vi "LinxI2cOpen.vi"(8 "Error In":errorcluster, 10 "I2C Channel":u8, 11 "LINX Resource":T1) -> (0 "Error Out":errorcluster, 3 "LINX Resource":T1)   [LabVIEW 2014, in "LMH-LINX.lvlib" / "Local IO.lvlib"]
uses:
  <vilib>/MakerHub/LINX/Private/Local IO/Local IO.lvlib
  <vilib>/MakerHub/LINX/Private/Type Defs/LINX Ref.ctl
  <vilib>/MakerHub/LINX/Private/Type Defs/Platform.ctl
  <vilib>/MakerHub/LINX/Private/Type Defs/Interface.ctl
  <vilib>/MakerHub/LINX/Private/Device/Type Defs/LINX Device Config.ctl
  <vilib>/MakerHub/LINX/Private/Device/Type Defs/TCP Config.ctl
  <vilib>/MakerHub/LINX/Private/Device/Type Defs/Channels.ctl
  <vilib>/MakerHub/LINX/Private/Type Defs/Channel FGV States.ctl
  <vilib>/myRIO/Instrument Drivers/Onboard IO/I2C/typedefs/I2C User Configuration.ctl
  <vilib>/myRIO/Instrument Drivers/Onboard IO/I2C/typedefs/I2C Transfer Rate.ctl
  <vilib>/Utility/error.llb/Error Cluster From Error Code.vi
  <vilib>/myRIO/Common/Instrument Driver Framework/myRIO v1.0/I2C/vis/myRIO v1.0 Configure I2C.vi
  <vilib>/MakerHub/LINX/LMH-LINX.lvlib
  <vilib>/MakerHub/LINX/Private/myRIO/myRIO.lvlib
  <vilib>/myRIO/Instrument Drivers/Onboard IO/I2C/I2C.lvlib
  liblinxdevice.dll
  <vilib>/MakerHub/LINX/Private/Device/Device.lvlib
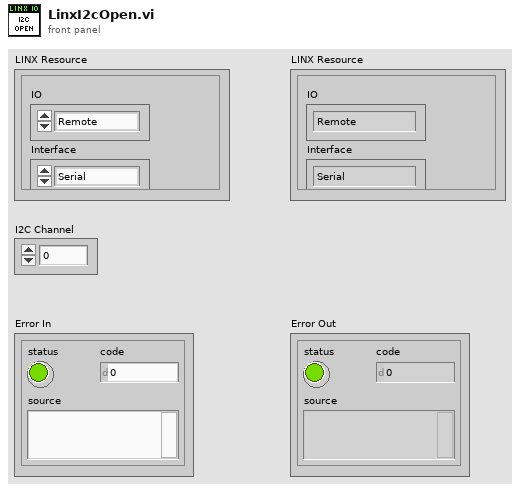
[diagram p1: front panel]
types:
  T1 = typedef "LMH-LINX.lvlib/LINX Ref.ctl" = cluster{"IO":T2, "Interface":T3, "LINX Device Config":T4}
  T2 = typedef "LMH-LINX.lvlib/Platform.ctl" = enum16{"Remote", "Local"}
  T3 = typedef "LMH-LINX.lvlib/Interface.ctl" = enum16{"Serial", "TCP"}
  T4 = typedef "LMH-LINX.lvlib/Device.lvlib/LINX Device Config.ctl" = cluster{"Interface":T3, "COM Port":refnum<visa-resource-name>, "TCP Configuration":T5, "Device Family":u8, "Device ID":u8, "Device Name":string, "TCP Ref":refnum<k5>, "Channels":T6}
  T5 = typedef "LMH-LINX.lvlib/Device.lvlib/TCP Config.ctl" = cluster{"IP Address":string, "Port":u16}
  T6 = typedef "LMH-LINX.lvlib/Channels.ctl" = cluster{"DI":u8[], "DO":u8[], "AI":u8[], "AO":u8[], "PWM":u8[], "QE":u8[], "UART":u8[], "I2C 2":u8[], "SPI":u8[], "CAN":u8[], "Servo":u8[], "AI Ref (V)":dbl, "AI Resolution (Bits)":u8, "AO Ref (V)":dbl, "AO Resolution (Bits)":u8}
  T7 = typedef "I2C.lvlib/I2C User Configuration.ctl" = cluster{"I2C Transfer Rate":T8}
  T8 = typedef "I2C.lvlib/I2C Transfer Rate.ctl" = enum16{"Standard mode (100 kbps)", "Fast mode (400 kbps)"}
  T9 = typedef "LMH-LINX.lvlib/Channel FGV States.ctl" = enum16{"Initialize", "Get", "Set"}
  T10 = typedef "I2C.lvlib/I2C Reference.ctl" = cluster{"myRIO Reference":T11, "I2C Channels Enum":T15, "I2C Configuration":T16}
  T11 = typedef "myRIO Generic Hardware Reference.ctl" = cluster{"myRIO Model":T12, "myRIO Hardware Reference":T13}
  T12 = typedef "Hardware Version Enum.ctl" = enum16{"Unknown", "myRIO-1900", "myRIO-1950"}
  T13 = typedef "myRIO v1.0 Reference.ctl" = cluster{"Generic FPGA Reference":T14, "Allow multiple opens":bool}
  T14 = typedef "Generic FPGA Reference.ctl" = refnum<k20>
  T15 = typedef "I2C Channels Enum.ctl" = enum16{"Not Connected", "A/I2C", "B/I2C"}
  T16 = typedef "I2C.lvlib/I2C Configuration.ctl" = cluster{"I2C Transfer Rate":T8}
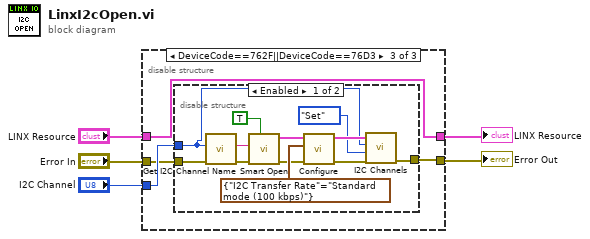
[diagram p0: block diagram]
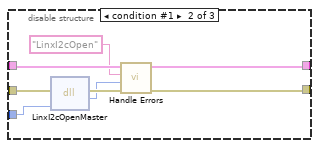
[diagram p3: hidden frame]
diagram:
  n1 = disable-structure shown="DeviceCode==762F||DeviceCode==76D3" {
    disable-tunnel: "LINX Resource" -> [w7 w14 w18]
    disable-tunnel: "Error In" -> [w6 w15 w16]
    disable-tunnel: [w6 w12 w19] -> w3
    disable-tunnel: [w7 w13 w18] -> w2
    disable-tunnel: "I2C Channel" -> [_ w8 w17]
    frame condition #0 {
    }
    frame condition #1 {
      n2 = dll-call lib="liblinxdevice.*" fn="LinxI2cOpenMaster"(error in=w15, "channel"=w8) -> (error out=w11:errorcluster, "LinxStatus"=w10:i32)  [unwired: 3 in, 1 out]
      n3 = call <vilib>:"Handle Errors.vi"("Error In"=w11, "LinxStatus"=w10, "Function Name"="LinxI2cOpen", "LINX Resource"=w14) -> ("Error Out"=w12:errorcluster, "LINX Resource"=w13:T1)  [unwired: 6 in]
    }
    frame condition #2 (active) {
      n4 = disable-structure shown="Enabled" {
        disable-tunnel: w16 -> [w21 w32]
        disable-tunnel: [w22 w32] -> w19
        disable-tunnel: w17 -> [w20 _]
        frame Enabled {
          n5 = call <vilib>:"Get I2C Channel Name.vi"("Error In"=w21, "I2C Channel"=w20) -> ("Error Out"=w29:errorcluster, "myRIO I2C Channels"=w28:string)  [unwired: 8 in]
          n6 = call <vilib>:"Smart Open.vi"("Allow multiple opens?"=TRUE, "error in (no error)"=w29, "Channel Name"=w28) -> ("error out"=w26:errorcluster, "I2C Ref Out"=w25:T10)  [unwired: 7 in]
          n7 = call <vilib>:"Configure.vi"("error in (no error)"=w26, "I2C User Configuration"=T7 {"I2C Transfer Rate"=enum."Standard mode (100 kbps)"}, "I2C Ref In"=w25) -> ("error out"=w31:errorcluster, "I2C Ref Out"=w30:T10)  [unwired: 7 in]
          n8 = call <vilib>:"I2C Channels.vi"("Error In"=w31, "Channel State"=Channel_FGV_States."Set", "Channel Number"=w20, "I2C Channel"=w30) -> ("Error Out"=w22:errorcluster)  [unwired: 6 in, 1 out]
        }
        frame Disabled {
          # "myRIO Support Disabled"
        }
      }
    }
  }
  "Error Out" <- w3
  "LINX Resource" <- w2
